vi "DataAcquisitionOpenClose.vi"(8 "error in (no error)":errorcluster, 10 "FilePath (Data Acquisition)":string, 11 "Open = true // Close = False":bool) -> (0 "error out":errorcluster)   [LabVIEW 2016]
uses:
  controls/Enum.ctl
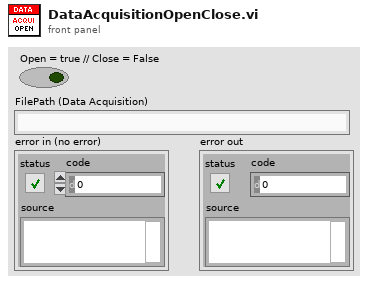
[diagram p1: front panel]
types:
  T1 = enum32{"Bad", "Idle", "Run top level", "Running"}
  T2 = typedef "Enum.ctl" = enum16{"Init", "Read", "Write"}
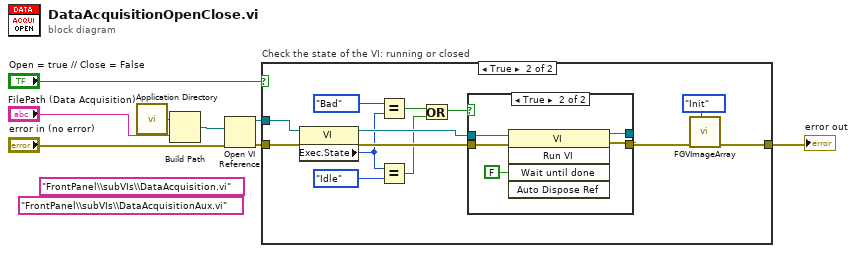
[diagram p0: block diagram]
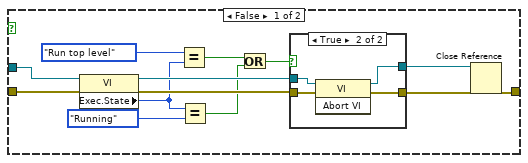
[diagram p2: hidden frame]
diagram:
  (unwired) "FrontPanel\\subVIs\\DataAcquisition.vi"
  (unwired) "FrontPanel\\subVIs\\DataAcquisitionAux.vi"
  n1 = call <vilib>:"Application Directory.vi"() -> ("Application Directory"=w6:path)
  n2 = Build Path(base path=w6, name or relative path="FilePath (Data Acquisition)") -> (appended path=w5:path)
  n3 = Open VI Reference(vi path=w5, error in (no error)="error in (no error)") -> (vi reference=w7:refnum<vi>, error out=w4:errorcluster)  [unwired: 4 in]
  n4 = case "Check the state of the VI: running or closed" shown="True" "Open = true // Close = False" {
    tunnel: w4 -> [w18 w37]
    tunnel: w7 -> [w11 w36]
    tunnel: [w10 w28] -> w1
    frame False {
      n5 = property class="VI"(reference=w11) -> (reference out=w19:refnum<vi>, "Exec.State"=w13:T1)  [unwired: 1 in, 1 out]
      n6 = Equal?(x=T1."Run top level" ("Execution:State"), y=w13) -> (x = y?=w15:bool)
      n7 = Equal?(x=w13, y=T1."Running" ("Execution:State")) -> (x = y?=w16:bool)
      n8 = Or(x=w15, y=w16) -> (x .or. y?=w17:bool)
      n9 = case shown="True" w17 {
        tunnel: [w21 w23] -> w10
        tunnel: w18 -> [w21 w25]
        tunnel: w19 -> [w20 w24]
        tunnel: [w20 w22] -> w9
        frame False {
        }
        frame True {
          n10 = invoke class="VI" method="Abort VI"(reference=w24, error in=w25) -> (reference out=w22:refnum<vi>, error out=w23:errorcluster)  [unwired: 1 in, 1 out]
        }
      }
      n11 = Close Reference(reference=w9) -> ()  [unwired: 1 in, 1 out]
    }
    frame True {
      n12 = property class="VI"(reference=w36) -> (reference out=w35:refnum<vi>, "Exec.State"=w33:T1)  [unwired: 1 in, 1 out]
      n13 = Equal?(x=T1."Bad" ("Execution:State"), y=w33) -> (x = y?=w31:bool)
      n14 = Equal?(x=w33, y=T1."Idle" ("Execution:State")) -> (x = y?=w30:bool)
      n15 = Or(x=w31, y=w30) -> (x .or. y?=w29:bool)
      n16 = case shown="True" w29 {
        tunnel: [w39 w41] -> w26
        tunnel: w37 -> [w39 w42]
        tunnel: w35 -> [w38 w43]
        tunnel: [w38 w40] -> _
        frame False {
        }
        frame True {
          n17 = invoke class="VI" method="Run VI"(reference=w43, error in=w42, "Wait until done"=FALSE ("Wait Until Done")) -> (reference out=w40:refnum<vi>, error out=w41:errorcluster)  [unwired: 2 in, 3 out]
        }
      }
      n18 = call "FGVImageArray.vi"("Enum"=Enum."Init", "error in"=w26) -> ("error out"=w28:errorcluster)  [unwired: 8 in, 1 out]
    }
  }
  "error out" <- w1
